vi "Read Data.vi"(8 "error in (no error)":errorcluster, 11 "Generic Update Data MSG in":refnum<class "Generic Update Data MSG.lvclass">) -> (0 "error out":errorcluster, 2 "Base Data Lib:Data":refnum<class "Data.lvclass">, 3 "Generic Update Data MSG out":refnum<class "Generic Update Data MSG.lvclass">)   [LabVIEW 2016, in "Generic Update Data MSG.lvclass"]
uses:
  Generic Update Data MSG.lvclass
  Data/Data.lvclass
  Generic Update Data MSG.lvclass/Generic Update Data MSG.ctl
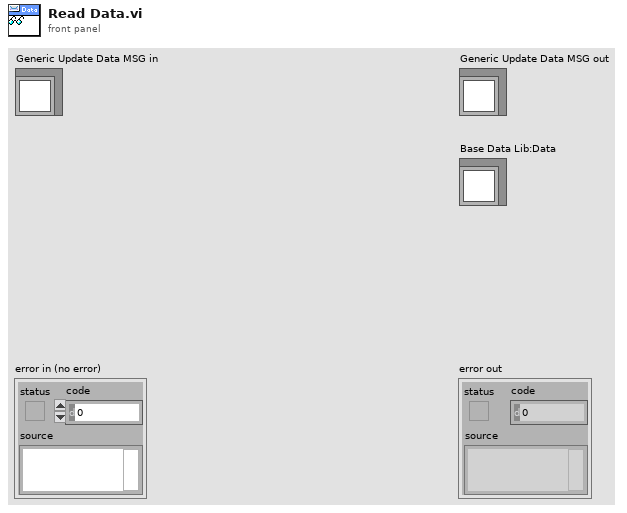
[diagram p1: front panel]
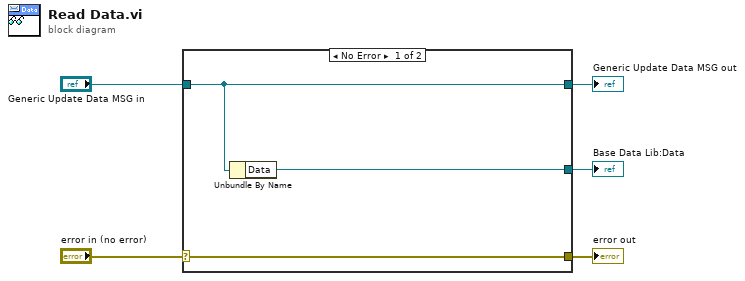
[diagram p0: block diagram]
diagram:
  n1 = case shown="No Error" "error in (no error)" {
    selector: "error in (no error)" -> [w8 w9]
    tunnel: [w8 w9] -> w4
    tunnel: [w7 w10] -> w2
    tunnel: "Generic Update Data MSG in" -> [w7 w10]
    tunnel: [w6 _] -> w1
    frame No Error {
      n2 = Unbundle By Name(w7) -> ("Data"=w6:refnum<class "Data.lvclass">)
    }
    frame Error {
    }
  }
  "error out" <- w4
  "Generic Update Data MSG out" <- w2
  "Base Data Lib:Data" <- w1
